vi "MatrixVg_Bdep&Tdep.vi"(3 "Time Stamp":timestamp, 6 "Play Button":bool) -> ()   [LabVIEW 2017]
uses:
  <vilib>/Utility/file.llb/Read From Spreadsheet File (DBL).vi
panel:
  in  "Custom Folder":string
  in  "T-table String":string
  out "T array":dbl[](array[numeric])
  in  "TCluster":T1={"Starting T (K)"=10.0, "Final T (K)"=20.0, "Step (K)"=1.0, "Time T stabilisation, min"=20.0, "After measurements"=TRUE} {"Final T (K)" min=-4.0 max=4.0 step=0.1 format="%.1f"; "Step (K)" min=0.0 max=1.0 step=0.01 format="%.1f"; "Starting T (K)" min=-4.0 max=4.0 step=0.1 format="%.1f"}
  out "Communication":string
  out "B Array":dbl[](array[numeric])
  in  "B-table String":string
  in  "BCluster":T2={"Starting B (T)"=-1.0, "Final B (T)"=1.0, "Step (T)"=1.0, "Time for persistant, min"=1.0} {"Final B (T)" min=-4.0 max=4.0 step=0.1 format="%.1f"; "Time for persistant, min" format="%.2f"; "Step (T)" min=0.0 max=1.0 step=0.01 format="%_4f"; "Starting B (T)" min=-4.0 max=4.0 step=0.1 format="%.1f"}
  out "Experiment ends at:":string
  out "Hours":dbl format="%.1f"
  out "Estimated time of experiment:":i16
  in  "Settings":T3={"Ring 3"=1, "Ring 2"=4, "Fixed Current mkA"=0.5, "If yes, the current is:"=enum."Radio Selection 1", "Ressitance measurements?"=TRUE, "Commute DC current?"=FALSE} {"Ring 3" items=["1 kOhm", "10 kOhm", "100 kOhm", "1 Mohm", "10 mOhm"]; "Ring 2" items=["1 kOhm", "10 kOhm", "100 kOhm", "1 Mohm", "10 MOhm"]}
  in  "Instruments":T4={"Oscillator"=TRUE, "Addr 1 lock-in"=TRUE, "Addr 1 lock-in oop"=TRUE, "Addr 2 lock-in"=FALSE, "Addr 2 lock-in oop"=FALSE, "Addr 3 lock-in"=FALSE, "Addr 3 lock-in oop"=FALSE, "Voltage (Vk1)"=FALSE, "Current (Ik1)"=TRUE, "Voltage (Vk2)"=FALSE, "Current (Ik2)"=FALSE, "Voltage (Vk3)"=FALSE, "Current (Ik3)"=FALSE, "Channel 1 (Vnano1)  "=FALSE, "Channel 2 (Vnano1b)"=FALSE, "Channel 1 (Vnano2)   "=FALSE, "Channel 2 (Vnano2b)"=FALSE, "Thermometer 1 (T1)"=TRUE, "Magnetic Field (B)"=TRUE, "Capacitance (C) and Loss (L)"=FALSE}
  in  "VgCluster":T5={"V1 (V)"=-1.0, "V2 (V)"=1.0, "Sweep rate, V/min"=1.0, "Time btw \npoints, sec"=1.0, "points at each Vg"=1, "Compliance, mkA"=0.05, "No-record rate, V/min"=30.0, "Full sweep?"=FALSE} {"No-record rate, V/min" min=0.0 max=1.0 step=0.01 format="%_4f"; "V2 (V)" min=-4.0 max=4.0 step=0.1 format="%.1f"; "Compliance, mkA" min=0.0 max=1.0 step=0.01 format="%.3f"; "Time btw \npoints, sec" format="%.2f"; "Sweep rate, V/min" min=0.0 max=1.0 step=0.01 format="%_4f"; "V1 (V)" min=-4.0 max=4.0 step=0.1 format="%.1f"}
  out "ArraySens":i8[](array[numeric])
  out "ArrayOsc":dbl[](array[numeric])
  out "# of configurations":i8
  out "Large Array":bool[][][](array[boolean])
  out "Contact configuration file (*.conf)":path
  # "hours"
  # "min.="
  # "Values of temperature can be also entered as the table by \ncopying and pasting a column of numbers in a \"T table\" \nstring at the far right side of this window."
  # "Values of B field can be also entered as the table by copying\nand pasting a column of numbers in a \"B table\" string at the \nfar right side of this window."
  # "Lock-in Amplifiers"
  # "Temperature"
  # "SourceMeters"
  # "Nanovoltmeters"
  # "Main"
  # "(not recommended, too slow)"
  # "Magnetic Field"
  # "Capacitance & Loss"
  # "(not recommended, too slow)"
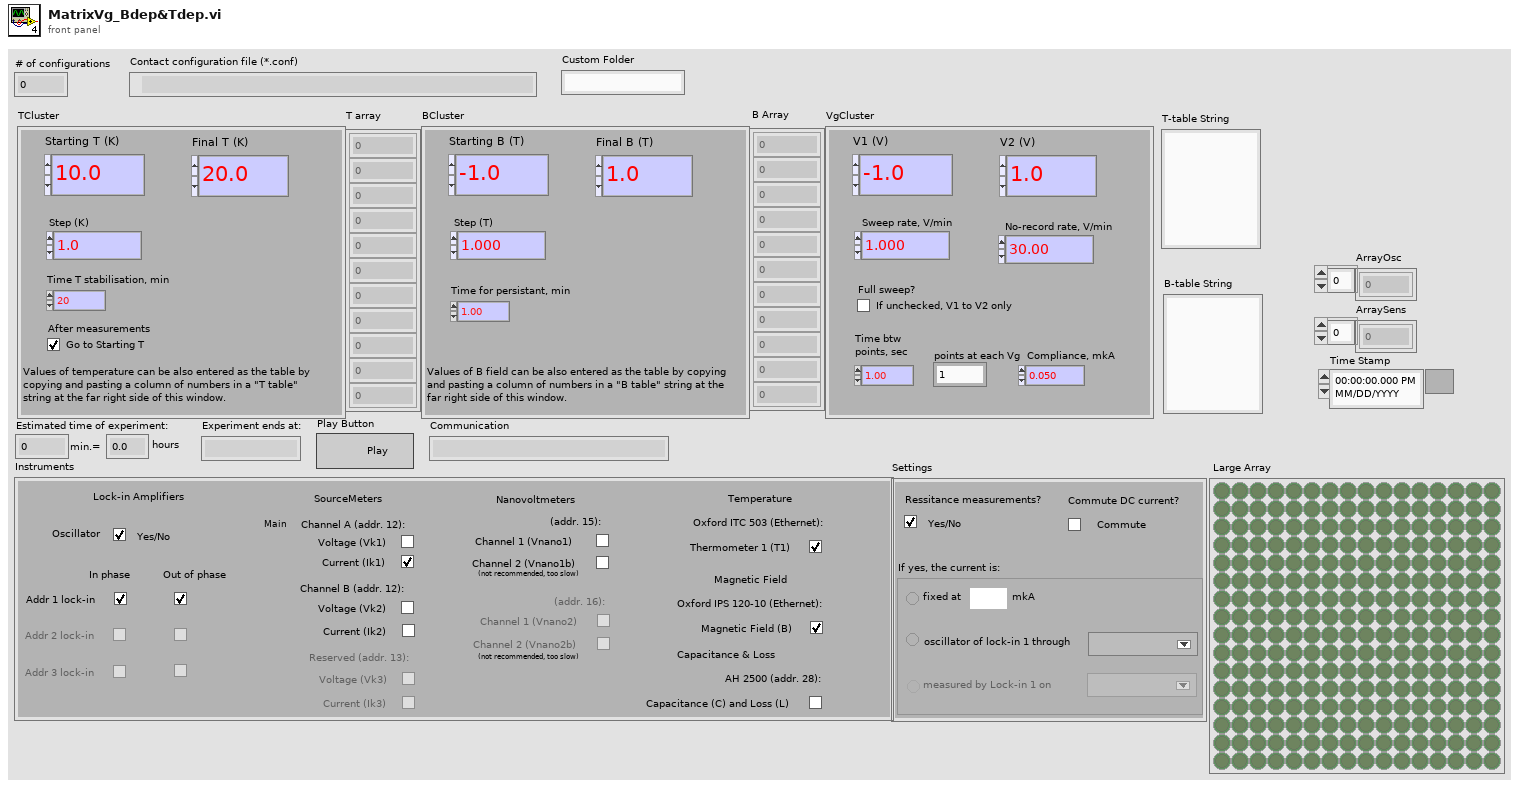
[diagram p1: front panel]
types:
  T1 = cluster{"Starting T (K)":dbl, "Final T (K)":dbl, "Step (K)":dbl, "Time T stabilisation, min":dbl, "After measurements":bool}
  T2 = cluster{"Starting B (T)":dbl, "Final B (T)":dbl, "Step (T)":dbl, "Time for persistant, min":dbl}
  T3 = cluster{"Ring 3":u16, "Ring 2":u16, "Fixed Current mkA":dbl, "If yes, the current is:":enum32{"Radio Selection 1", "Radio Selection 2", "Radio Selection 3"}, "Ressitance measurements?":bool, "Commute DC current?":bool}
  T4 = cluster{"Oscillator":bool, "Addr 1 lock-in":bool, "Addr 1 lock-in oop":bool, "Addr 2 lock-in":bool, "Addr 2 lock-in oop":bool, "Addr 3 lock-in":bool, "Addr 3 lock-in oop":bool, "Voltage (Vk1)":bool, "Current (Ik1)":bool, "Voltage (Vk2)":bool, "Current (Ik2)":bool, "Voltage (Vk3)":bool, "Current (Ik3)":bool, "Channel 1 (Vnano1)  ":bool, "Channel 2 (Vnano1b)":bool, "Channel 1 (Vnano2)   ":bool, "Channel 2 (Vnano2b)":bool, "Thermometer 1 (T1)":bool, "Magnetic Field (B)":bool, "Capacitance (C) and Loss (L)":bool}
  T5 = cluster{"V1 (V)":dbl, "V2 (V)":dbl, "Sweep rate, V/min":dbl, "Time btw \npoints, sec":dbl, "points at each Vg":i32, "Compliance, mkA":dbl, "No-record rate, V/min":dbl, "Full sweep?":bool}
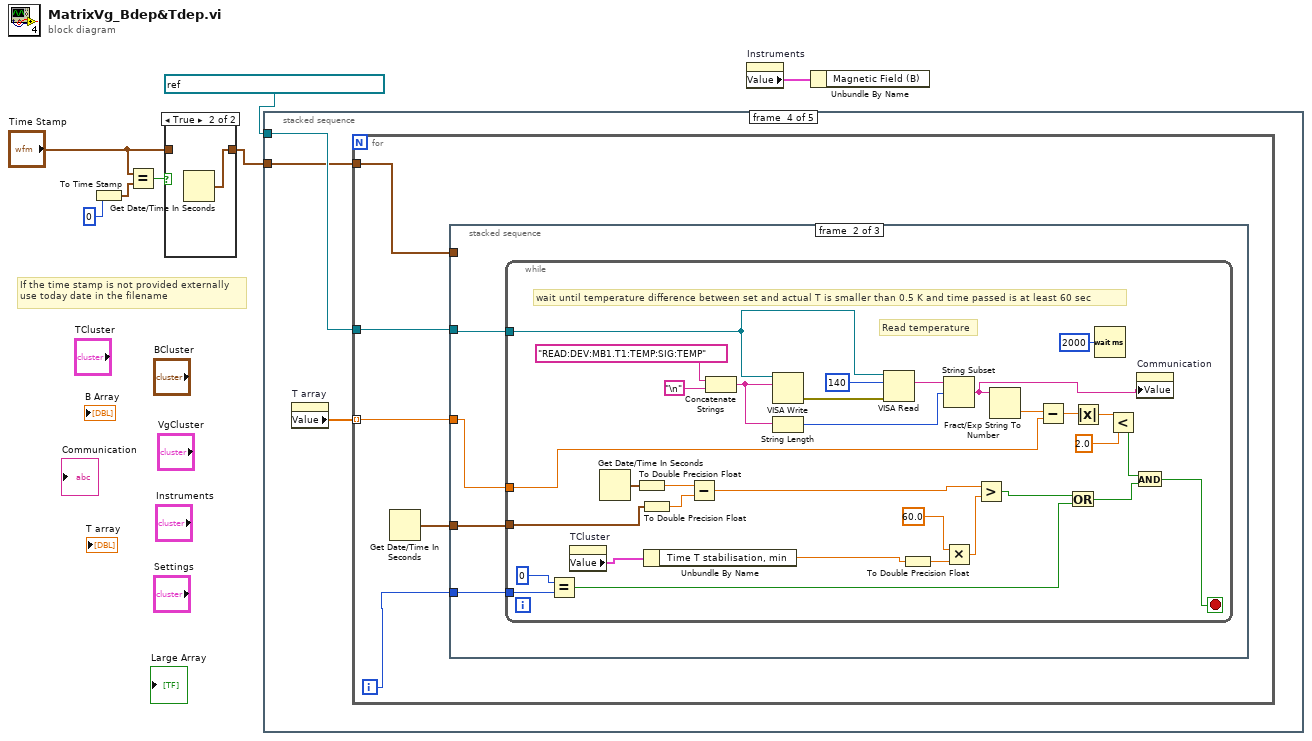
[diagram p0: block diagram]
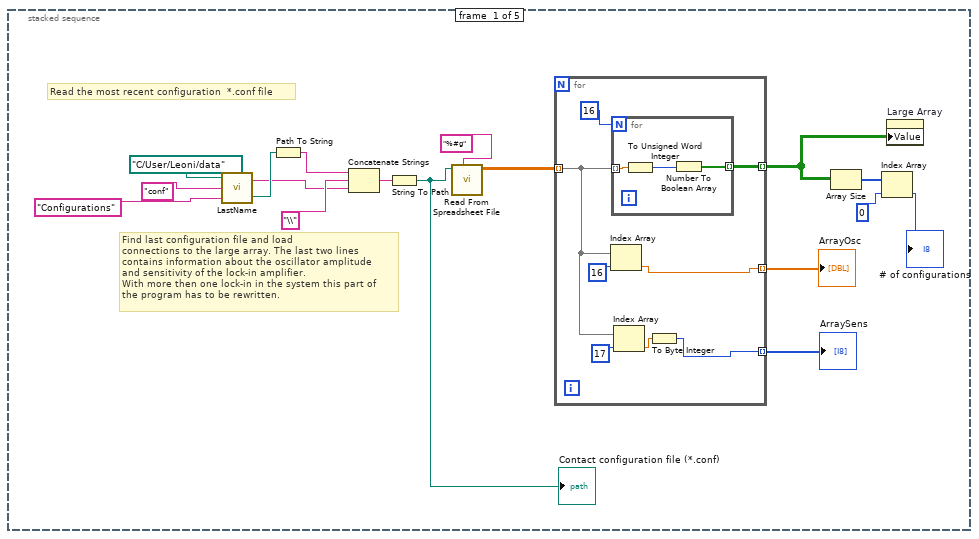
[diagram p3: hidden frame]
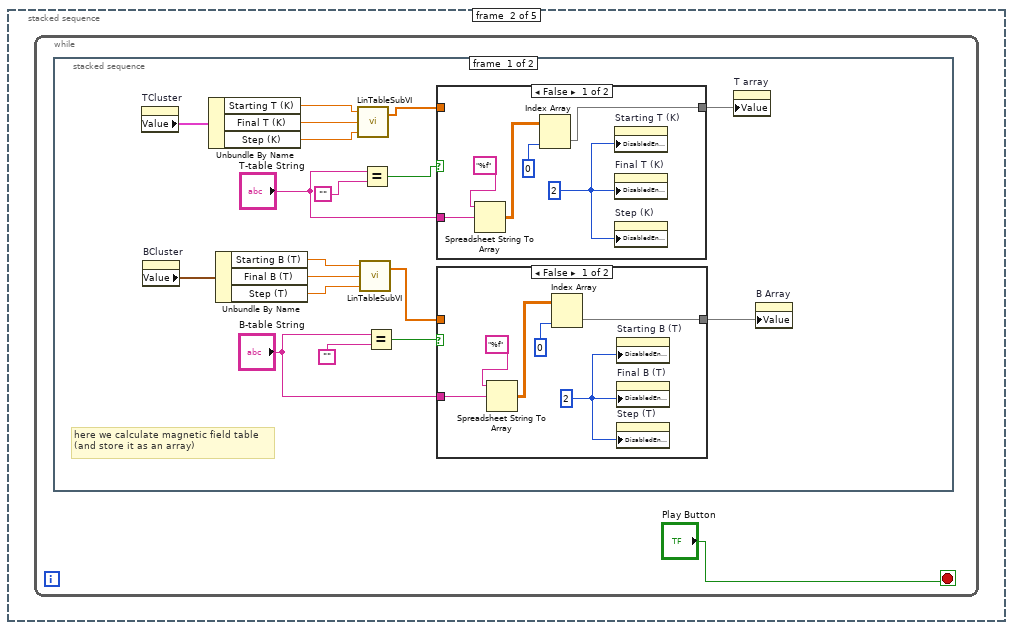
[diagram p4: hidden frame]
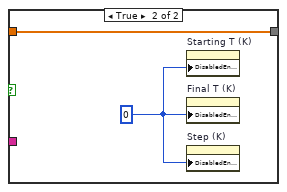
[diagram p5: hidden frame]
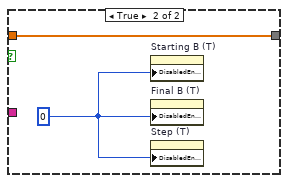
[diagram p6: hidden frame]
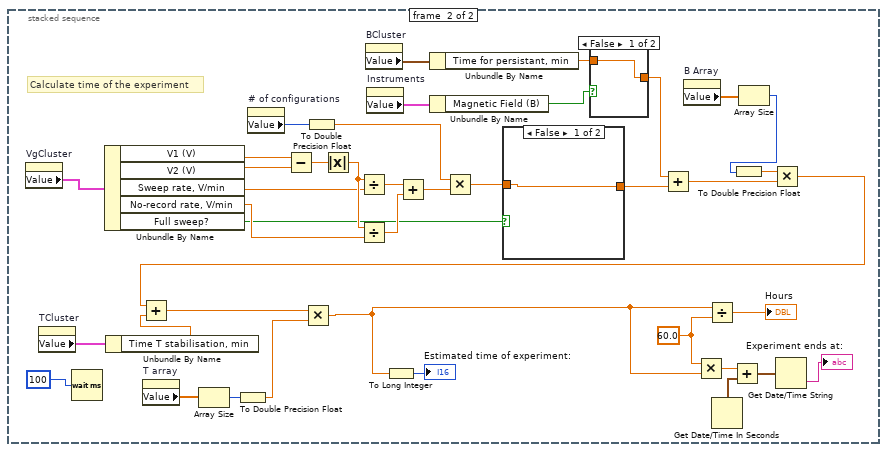
[diagram p7: hidden frame]
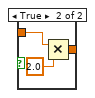
[diagram p8: hidden frame]
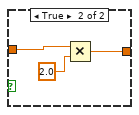
[diagram p9: hidden frame]
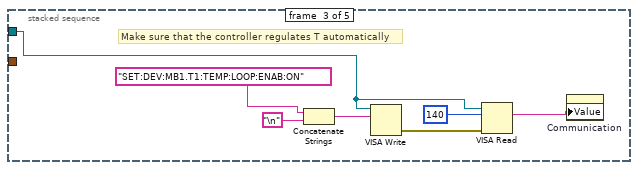
[diagram p10: hidden frame]
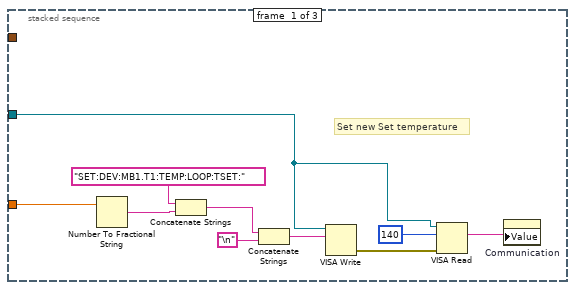
[diagram p11: hidden frame]
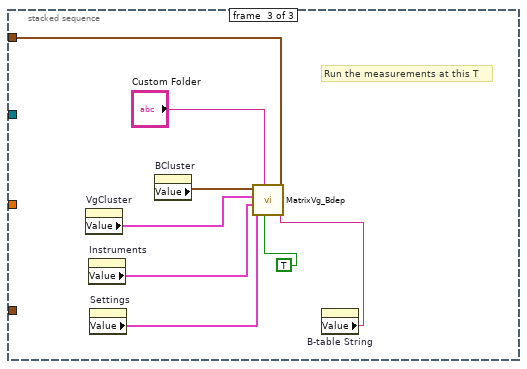
[diagram p12: hidden frame]
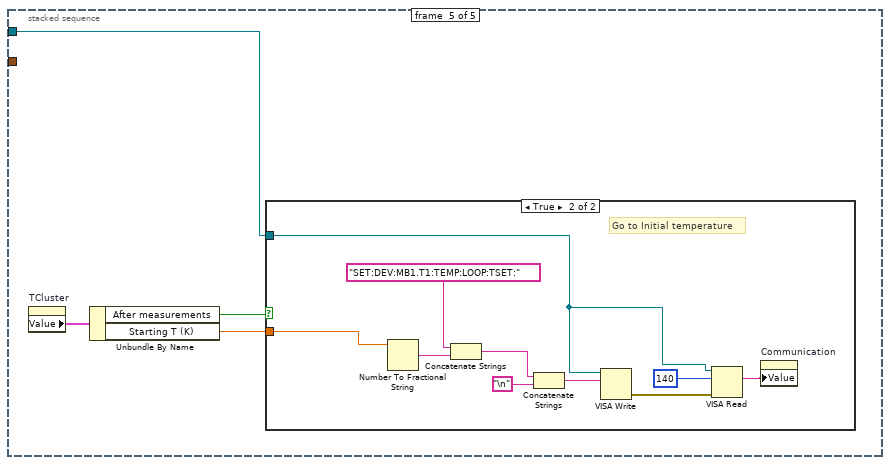
[diagram p13: hidden frame]
diagram:
  # "If the time stamp is not provided externally\nuse today date in the filename"
  n1 = To Time Stamp(1:0) -> (0:w6:timestamp)
  n2 = Equal?(x="Time Stamp", y=w6) -> (x = y?=w5:bool)
  n3 = case shown="True" w5 {
    tunnel: "Time Stamp" -> [w8 _]
    tunnel: [w8 w9] -> w3
    frame False {
    }
    frame True {
      n4 = Get Date/Time In Seconds() -> (seconds since 1Jan1904=w9:timestamp)
    }
  }
  n5 = stacked-sequence {
    tunnel: w3 -> [_ _ _ w129 _]
    tunnel: refnum<visa-resource-name> "TCPIP0::192.168.128.2::7020::SOCKET" ("VISA resource name") -> [_ _ w122 w130 w191]
    frame #0 {
      # "Read the most recent configuration  *.conf file"
      # "Find last configuration file and load \nconnections to the large array. The last two lines \ncontains information about the oscillator amplitude\nand sensitivity of the lock-in amplifier.\nWith more then one lock-in in the system this part of \nthe program has to be rewritten."
      n6 = call "LastName.vi"("Custom Folder"="Configurations", "Extention"="conf", "User Data Folder"=path "C:/User/Leoni/data") -> ("created path"=w22:path, "String"=w21:string)
      n7 = Path To String(path=w22) -> (string=w26:string)
      n8 = Concatenate Strings(w26, "\\", w21) -> (w24:string)
      n9 = String To Path(string=w24) -> (path=w12:path)
      "Contact configuration file (*.conf)" <- w12
      n10 = call-poly <vilib>:"Read From Spreadsheet File.vi"("format (%.3f)"="%#g", "file path (dialog if empty)"=w12) -> ("all rows"=w17:dbl[][])  [unwired: 5 in, 4 out]
      n11 = for {
        tunnel: w17 -> [w30] mode=indexing
        tunnel: [w34] -> w14 mode=indexing
        tunnel: [w29] -> w11 mode=indexing
        tunnel: [w28] -> w10 mode=indexing
        n12 = Index Array(array=w30, index=16) -> (element=w29:dbl)
        n13 = for {
          N: 16 -> [_]
          tunnel: w30 -> [w37] mode=indexing
          tunnel: [w35] -> w34 mode=indexing
          n14 = To Unsigned Word Integer(number=w37) -> (unsigned 16bit integer=w36:u16)
          n15 = Number To Boolean Array(number=w36) -> (Boolean array=w35:bool[])
        }
        n16 = Index Array(array=w30, index=17) -> (element=w31:dbl)
        n17 = To Byte Integer(number=w31) -> (8bit integer=w28:i8)
      }
      "ArrayOsc" <- w11
      "ArraySens" <- w10
      n18 = Array Size(array=w14) -> (size(s)=w16:i32[])
      n19 = Index Array(array=w16, index=0) -> (element=→"# of configurations":i32)
      n20 = property on="Large Array" class="Arr (strict)"("Value"=w14) -> ()  [unwired: 2 in, 2 out]
    }
    frame #1 {
      n21 = while {
        stop <- "Play Button" stop-if-true
        n22 = stacked-sequence {
          frame #0 {
            # "here we calculate magnetic field table\n(and store it as an array)"
            n23 = property on="TCluster" class="Clust (strict)"() -> ("Value"=w47:T1)  [unwired: 2 in, 2 out]
            n24 = property on="BCluster" class="Clust (strict)"() -> ("Value"=w52:T2)  [unwired: 2 in, 2 out]
            n25 = Unbundle By Name(w47) -> ("Starting T (K)"=w46:dbl, "Final T (K)"=w45:dbl, "Step (K)"=w44:dbl)
            n26 = Unbundle By Name(w52) -> ("Starting B (T)"=w51:dbl, "Final B (T)"=w50:dbl, "Step (T)"=w49:dbl)
            n27 = call "LinTableSubVI.vi"("Step"=w44, "Final"=w45, "Initial"=w46) -> ("Array"=w40:dbl[])  [unwired: 1 in]
            n28 = call "LinTableSubVI.vi"("Step"=w49, "Final"=w50, "Initial"=w51) -> ("Array"=w56:dbl[])  [unwired: 1 in]
            n29 = Equal?(x="T-table String", y="") -> (x = y?=w42:bool)
            n30 = Equal?(x="B-table String", y="") -> (x = y?=w53:bool)
            n31 = case shown="False" w42 {
              tunnel: [w58 w63] -> w41
              tunnel: w40 -> [_ w63]
              tunnel: "T-table String" -> [w57 _]
              frame False {
                w59 = 2
                n32 = Spreadsheet String To Array(format string="%f", spreadsheet string=w57) -> (array=w61:dbl[][])  [unwired: 2 in]
                n33 = Index Array(array=w61, index (col)=0) -> (element=w58:dbl[])  [unwired: 1 in]
                n34 = property on="Starting T (K)" class="DigNum (strict)"("DisabledEnum"=w59) -> ()  [unwired: 2 in, 2 out]
                n35 = property on="Final T (K)" class="DigNum (strict)"("DisabledEnum"=w59) -> ()  [unwired: 2 in, 2 out]
                n36 = property on="Step (K)" class="DigNum (strict)"("DisabledEnum"=w59) -> ()  [unwired: 2 in, 2 out]
              }
              frame True {
                w64 = 0
                n37 = property on="Starting T (K)" class="DigNum (strict)"("DisabledEnum"=w64) -> ()  [unwired: 2 in, 2 out]
                n38 = property on="Final T (K)" class="DigNum (strict)"("DisabledEnum"=w64) -> ()  [unwired: 2 in, 2 out]
                n39 = property on="Step (K)" class="DigNum (strict)"("DisabledEnum"=w64) -> ()  [unwired: 2 in, 2 out]
              }
            }
            n40 = case shown="False" w53 {
              tunnel: [w67 w72] -> w48
              tunnel: w56 -> [_ w72]
              tunnel: "B-table String" -> [w66 _]
              frame False {
                w65 = 2
                n41 = Spreadsheet String To Array(format string="%f", spreadsheet string=w66) -> (array=w69:dbl[][])  [unwired: 2 in]
                n42 = Index Array(array=w69, index (col)=0) -> (element=w67:dbl[])  [unwired: 1 in]
                n43 = property on="Starting B (T)" class="DigNum (strict)"("DisabledEnum"=w65) -> ()  [unwired: 2 in, 2 out]
                n44 = property on="Final B (T)" class="DigNum (strict)"("DisabledEnum"=w65) -> ()  [unwired: 2 in, 2 out]
                n45 = property on="Step (T)" class="DigNum (strict)"("DisabledEnum"=w65) -> ()  [unwired: 2 in, 2 out]
              }
              frame True {
                w71 = 0
                n46 = property on="Starting B (T)" class="DigNum (strict)"("DisabledEnum"=w71) -> ()  [unwired: 2 in, 2 out]
                n47 = property on="Final B (T)" class="DigNum (strict)"("DisabledEnum"=w71) -> ()  [unwired: 2 in, 2 out]
                n48 = property on="Step (T)" class="DigNum (strict)"("DisabledEnum"=w71) -> ()  [unwired: 2 in, 2 out]
              }
            }
            n49 = property on="T array" class="Arr (strict)"("Value"=w41) -> ()  [unwired: 2 in, 2 out]
            n50 = property on="B Array" class="Arr (strict)"("Value"=w48) -> ()  [unwired: 2 in, 2 out]
          }
          frame #1 {
            w92 = 60.0
            # "Calculate time of the experiment"
            n51 = property on="VgCluster" class="Clust (strict)"() -> ("Value"=w111:T5)  [unwired: 2 in, 2 out]
            n52 = property on="TCluster" class="Clust (strict)"() -> ("Value"=w80:T1)  [unwired: 2 in, 2 out]
            n53 = Wait (ms)(milliseconds to wait=100) -> ()  [unwired: 1 out]
            n54 = Unbundle By Name(w111) -> ("V1 (V)"=w110:dbl, "V2 (V)"=w109:dbl, "Sweep rate, V/min"=w106:dbl, "No-record rate, V/min"=w105:dbl, "Full sweep?"=w99:bool)
            n55 = Unbundle By Name(w80) -> ("Time T stabilisation, min"=w78:dbl)
            n56 = property on="T array" class="Arr (strict)"() -> ("Value"=w77:dbl[])  [unwired: 2 in, 2 out]
            n57 = Array Size(array=w77) -> (size(s)=w76:i32)
            n58 = To Double Precision Float(number=w76) -> (double precision float=w75:dbl)
            n59 = property on="# of configurations" class="DigNum (strict)"() -> ("Value"=w101:i8)  [unwired: 2 in, 2 out]
            n60 = Subtract(x=w110, y=w109) -> (x-y=w108:dbl)
            n61 = To Double Precision Float(number=w101) -> (double precision float=w100:dbl)
            n62 = Absolute Value(x=w108) -> (abs(x)=w107:dbl)
            n63 = Divide(x=w107, y=w106) -> (x/y=w104:dbl)
            n64 = Divide(x=w107, y=w105) -> (x/y=w103:dbl)
            n65 = property on="BCluster" class="Clust (strict)"() -> ("Value"=w88:T2)  [unwired: 2 in, 2 out]
            n66 = property on="Instruments" class="Clust (strict)"() -> ("Value"=w84:T4)  [unwired: 2 in, 2 out]
            n67 = Add(x=w104, y=w103) -> (x+y=w102:dbl)
            n68 = Unbundle By Name(w88) -> ("Time for persistant, min"=w82:dbl)
            n69 = Unbundle By Name(w84) -> ("Magnetic Field (B)"=w83:bool)
            n70 = Multiply(x=w100, y=w102) -> (x*y=w98:dbl)
            n71 = case shown="False" w99 {
              tunnel: w98 -> [w117 w120]
              tunnel: [w117 w118] -> w89
              frame False {
              }
              frame True {
                n72 = Multiply(x=w120, y=2.0) -> (x*y=w118:dbl)
              }
            }
            n73 = case shown="False" w83 {
              tunnel: w82 -> [w113 w115]
              tunnel: [w113 w114] -> w81
              frame False {
              }
              frame True {
                n74 = Multiply(x=w115, y=2.0) -> (x*y=w114:dbl)
              }
            }
            n75 = Add(x=w81, y=w89) -> (x+y=w87:dbl)
            n76 = property on="B Array" class="Arr (strict)"() -> ("Value"=w90:dbl[])  [unwired: 2 in, 2 out]
            n77 = Get Date/Time In Seconds() -> (seconds since 1Jan1904=w96:timestamp)
            n78 = Array Size(array=w90) -> (size(s)=w85:i32)
            n79 = To Double Precision Float(number=w85) -> (double precision float=w86:dbl)
            n80 = Multiply(x=w86, y=w87) -> (x*y=w79:dbl)
            n81 = Add(x=w79, y=w78) -> (x+y=w74:dbl)
            n82 = Multiply(x=w74, y=w75) -> (x*y=w73:dbl)
            n83 = To Long Integer(number=w73) -> (32bit integer=→"Estimated time of experiment:":i32)
            n84 = Multiply(x=w92, y=w73) -> (x*y=w91:dbl)
            n85 = Divide(x=w73, y=w92) -> (x/y=→"Hours":dbl)
            n86 = Add(x=w91, y=w96) -> (x+y=w95:timestamp)
            n87 = Get Date/Time String(seconds (now)=w95) -> (time string=→"Experiment ends at:":string)  [unwired: 2 in, 1 out]
          }
        }
      }
    }
    frame #2 {
      # "Make sure that the controller regulates T automatically"
      n88 = Concatenate Strings("SET:DEV:MB1.T1:TEMP:LOOP:ENAB:ON" ("string"), "\n") -> (w124:string)
      n89 = VISA Write(VISA resource name=w122, write buffer=w124) -> (error out=w127:errorcluster)  [unwired: 1 in, 2 out]
      n90 = VISA Read(VISA resource name=w122, byte count=140, error in (no error)=w127) -> (read buffer=w121:string)  [unwired: 3 out]
      n91 = property on="Communication" class="Str"("Value"=w121) -> ()  [unwired: 2 in, 2 out]
    }
    frame #3 {
      n92 = property on="T array" class="Arr (strict)"() -> ("Value"=w128:dbl[])  [unwired: 2 in, 2 out]
      n93 = for {
        tunnel: w130 -> [w135]
        tunnel: w128 -> [w134] mode=indexing
        tunnel: w129 -> [w132]
        i -> [w131]
        n94 = Get Date/Time In Seconds() -> (seconds since 1Jan1904=w133:timestamp)
        n95 = stacked-sequence {
          tunnel: w135 -> [w138 w149 _]
          tunnel: w134 -> [w136 w148 _]
          tunnel: w133 -> [_ w147 _]
          tunnel: w132 -> [_ _ w184]
          tunnel: w131 -> [_ w146 _]
          frame #0 {
            # "Set new Set temperature"
            n96 = Number To Fractional String(number=w136) -> (F-format string=w140:string)  [unwired: 3 in]
            n97 = Concatenate Strings("SET:DEV:MB1.T1:TEMP:LOOP:TSET:" ("string"), w140) -> (w145:string)
            n98 = Concatenate Strings(w145, "\n") -> (w144:string)
            n99 = VISA Write(VISA resource name=w138, write buffer=w144) -> (error out=w141:errorcluster)  [unwired: 1 in, 2 out]
            n100 = VISA Read(VISA resource name=w138, byte count=140, error in (no error)=w141) -> (read buffer=w137:string)  [unwired: 3 out]
            n101 = property on="Communication" class="Str"("Value"=w137) -> ()  [unwired: 2 in, 2 out]
          }
          frame #1 {
            n102 = while {
              tunnel: w149 -> [w174]
              tunnel: w148 -> [w172]
              tunnel: w147 -> [w167]
              tunnel: w146 -> [w150]
              stop <- w162 stop-if-true
              # "wait until temperature difference between set and actual T is smaller than 0.5 K and time passed is at least 60 sec"
              # "Read temperature"
              n103 = Equal?(x=0, y=w150) -> (x = y?=w158:bool)
              n104 = property on="TCluster" class="Clust (strict)"() -> ("Value"=w152:T1)  [unwired: 2 in, 2 out]
              n105 = Get Date/Time In Seconds() -> (seconds since 1Jan1904=w168:timestamp)
              n106 = To Double Precision Float(number=w168) -> (double precision float=w166:dbl)
              n107 = To Double Precision Float(number=w167) -> (double precision float=w165:dbl)
              n108 = Unbundle By Name(w152) -> ("Time T stabilisation, min"=w151:dbl)
              n109 = Subtract(x=w166, y=w165) -> (x-y=w164:dbl)
              n110 = Concatenate Strings("READ:DEV:MB1.T1:TEMP:SIG:TEMP" ("string"), "\n") -> (w175:string)
              n111 = VISA Write(VISA resource name=w174, write buffer=w175) -> (error out=w181:errorcluster)  [unwired: 1 in, 2 out]
              n112 = String Length(string=w175) -> (length=w176:i32)
              n113 = VISA Read(VISA resource name=w174, byte count=140, error in (no error)=w181) -> (read buffer=w177:string)  [unwired: 3 out]
              n114 = To Double Precision Float(number=w151) -> (double precision float=w156:dbl)
              n115 = String Subset(string=w177, offset (0)=w176) -> (substring=w153:string)  [unwired: 1 in]
              n116 = Multiply(x=60.0, y=w156) -> (x*y=w154:dbl)
              n117 = Greater?(x=w164, y=w154) -> (0:w159:bool)
              n118 = Fract/Exp String To Number(string=w153) -> (number=w173:dbl)  [unwired: 3 in, 1 out]
              n119 = Subtract(x=w173, y=w172) -> (x-y=w171:dbl)
              n120 = Or(x=w159, y=w158) -> (x .or. y?=w157:bool)
              n121 = Absolute Value(x=w171) -> (abs(x)=w170:dbl)
              n122 = Wait (ms)(milliseconds to wait=2000) -> ()  [unwired: 1 out]
              n123 = Less?(x=w170, y=2.0) -> (x < y?=w163:bool)
              n124 = And(x=w163, y=w157) -> (x .and. y?=w162:bool)
              n125 = property on="Communication" class="Str"("Value"=w153) -> ()  [unwired: 2 in, 2 out]
            }
          }
          frame #2 {
            # "Run the measurements at this T"
            n126 = property on="VgCluster" class="Clust (strict)"() -> ("Value"=w188:T5)  [unwired: 2 in, 2 out]
            n127 = property on="Instruments" class="Clust (strict)"() -> ("Value"=w187:T4)  [unwired: 2 in, 2 out]
            n128 = property on="Settings" class="Clust (strict)"() -> ("Value"=w186:T3)  [unwired: 2 in, 2 out]
            n129 = property on="BCluster" class="Clust (strict)"() -> ("Value"=w189:T2)  [unwired: 2 in, 2 out]
            n130 = property on="B-table String" class="Str"() -> ("Value"=w183:string)  [unwired: 2 in, 2 out]
            n131 = call "MatrixVg_Bdep.vi"("B-table String"=w183, "Time Stamp"=w184, "Play Button"=TRUE, "Custom Folder"="Custom Folder", "Settings"=w186, "Instruments"=w187, "VgCluster"=w188, "BCluster"=w189) -> ()  [unwired: 4 in]
          }
        }
      }
    }
    frame #4 {
      n132 = property on="TCluster" class="Clust (strict)"() -> ("Value"=w193:T1)  [unwired: 2 in, 2 out]
      n133 = Unbundle By Name(w193) -> ("After measurements"=w192:bool, "Starting T (K)"=w190:dbl)
      n134 = case shown="True" w192 {
        tunnel: w191 -> [_ w196]
        tunnel: w190 -> [_ w194]
        frame False {
          # "Stay at current T"
        }
        frame True {
          # "Go to Initial temperature"
          n135 = Number To Fractional String(number=w194) -> (F-format string=w198:string)  [unwired: 3 in]
          n136 = Concatenate Strings("SET:DEV:MB1.T1:TEMP:LOOP:TSET:" ("string"), w198) -> (w203:string)
          n137 = Concatenate Strings(w203, "\n") -> (w202:string)
          n138 = VISA Write(VISA resource name=w196, write buffer=w202) -> (error out=w199:errorcluster)  [unwired: 1 in, 2 out]
          n139 = VISA Read(VISA resource name=w196, byte count=140, error in (no error)=w199) -> (read buffer=w195:string)  [unwired: 3 out]
          n140 = property on="Communication" class="Str"("Value"=w195) -> ()  [unwired: 2 in, 2 out]
        }
      }
    }
  }
  n141 = property on="Instruments" class="Clust (strict)"() -> ("Value"=w1:T4)  [unwired: 2 in, 2 out]
  n142 = Unbundle By Name(w1) -> ()  [unwired: 1 out]
